vi "Wait for Operation Complete.vi"(8 "error in (no error)":errorcluster, 10 "Timeout (10000 ms)":u32=10000, 11 "VISA resource name":refnum<visa-resource-name>) -> (0 "error out":errorcluster, 3 "VISA resource name out":refnum<visa-resource-name>)   [LabVIEW 2018, in "Keithley 24XX.lvlib"]
doc: "Waits for an operation to complete. This is useful for synchronizing instrument code with other code.\n\n<B>Note:</B> When taking measurements, this VI will hold until the instrument has armed and triggered all of the times specified in Configure Multipoint. This VI won't function correctly if the triggering has occured but the instrument is set to arm after those triggered measurements have finished.\n\nUse this VI only with other low-level VIs. The high-level VIs automatically incorporate this functionality. This VI does not check the instrument status. If you want to check the instrument status, call the Error Query VI at the conclusion of the sequence."
uses:
  Keithley 24XX.lvlib
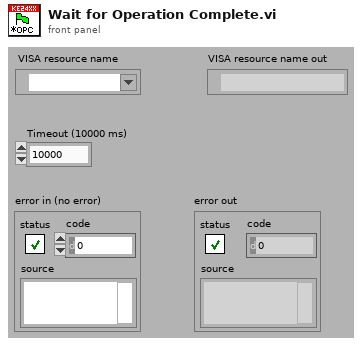
[diagram p1: front panel]
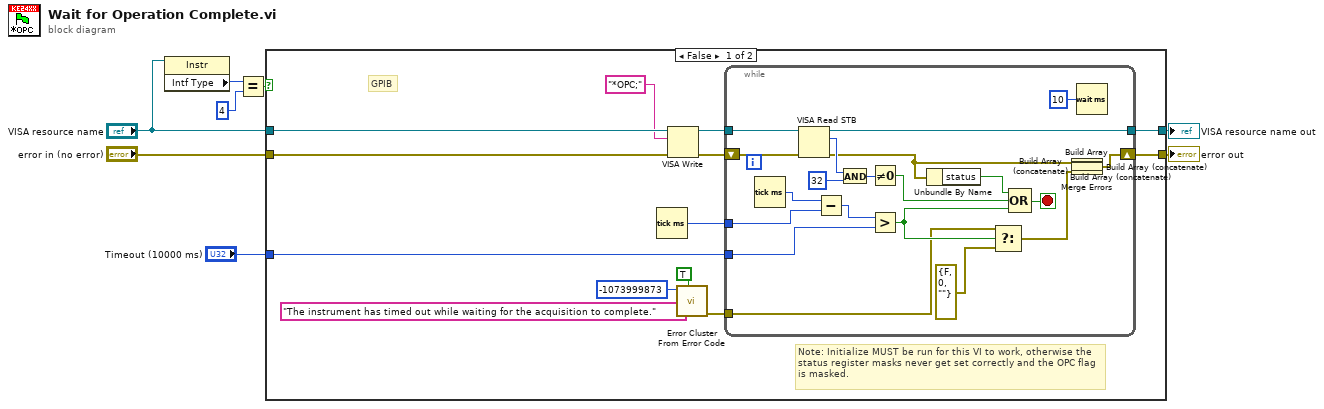
[diagram p0: block diagram]
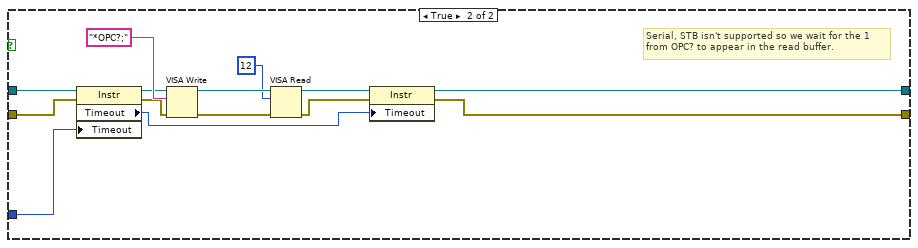
[diagram p2: hidden frame]
diagram:
  n1 = property class="Instr"(reference="VISA resource name") -> ("Intf Type"=w3:u16)  [unwired: 1 in, 2 out]
  n2 = Equal?(x=w3, y=u16 4) -> (x = y?=w4:bool)
  n3 = case shown="False" w4 {
    tunnel: "VISA resource name" -> [w21 w55]
    tunnel: "error in (no error)" -> [w20 w50]
    tunnel: [w17 w46] -> w7
    tunnel: [w16 w51] -> w6
    tunnel: "Timeout (10000 ms)" -> [w9 w54]
    frame False {
      # "GPIB"
      # "Note: Initialize MUST be run for this VI to work, otherwise the status register masks never get set correctly and the OPC flag is masked."
      n4 = Tick Count (ms)() -> (millisecond timer value=w14:u32)
      n5 = VISA Write(VISA resource name=w21, write buffer="*OPC;", error in (no error)=w20) -> (VISA resource name out=w19:refnum<visa-resource-name>, error out=w18:errorcluster)  [unwired: 1 out]
      n6 = call <vilib>:"Error Cluster From Error Code.vi"("show call chain? (False)"=TRUE, "error message (\"\")"="The instrument has timed out while waiting for the acquisition to complete." ("error message (\"\")"), "error code (0)"=-1073999873) -> ("error out"=w10:errorcluster)  [unwired: 6 in]
      n7 = while {
        tunnel: w19 -> [w45]
        tunnel: [w43] -> w16
        tunnel: w14 -> [w38]
        shift-right: [w30] -> w17
        shift-left: w18 -> [w44]
        tunnel: w10 -> [w33]
        tunnel: w9 -> [w26]
        stop <- w35 stop-if-true
        n8 = Tick Count (ms)() -> (millisecond timer value=w39:u32)
        n9 = VISA Read STB(8:w44, 11:w45) -> (0:w29:errorcluster, 2:w42:u16, 3:w43:refnum<visa-resource-name>)
        n10 = Subtract(x=w39, y=w38) -> (x-y=w37:u32)
        n11 = And(x=w42, y=u16 32) -> (x .and. y?=w40:u16)
        n12 = Not Equal To 0?(x=w40) -> (x != 0?=w36:bool)
        n13 = Greater?(x=w37, y=w26) -> (0:w34:bool)
        n14 = Unbundle By Name(w29) -> ("status"=w28:bool)
        n15 = Select(t=w33, s=w34, f=errorcluster {"status"=FALSE, "code"=0, "source"=""}) -> (s? t:f=w31:errorcluster)
        n16 = Compound Arithmetic op=OR(w28, w36, w34) -> (w35:bool)
        n17 = Build Array(w29, w31) -> (w25:errorcluster[])
        n18 = Build Array (concatenate)(w25) -> (w24:errorcluster[])
        n19 = Build Array (concatenate)(w24) -> (w23:errorcluster[])
        n20 = Build Array (concatenate)(w23) -> (w22:errorcluster[])
        n21 = Merge Errors(w22) -> (w30:errorcluster)
        n22 = Wait (ms)(milliseconds to wait=u32 10) -> ()  [unwired: 1 out]
      }
    }
    frame True {
      # "Serial, STB isn't supported so we wait for the 1 \nfrom OPC? to appear in the read buffer."
      n23 = property class="Instr"(reference=w55, error in=w50, "Timeout"=w54) -> (reference out=w49:refnum<visa-resource-name>, error out=w48:errorcluster, "Timeout"=w53:u32)
      n24 = VISA Write(VISA resource name=w49, write buffer="*OPC?;", error in (no error)=w48) -> (VISA resource name out=w57:refnum<visa-resource-name>, error out=w58:errorcluster)  [unwired: 1 out]
      n25 = VISA Read(VISA resource name=w57, byte count=u32 12, error in (no error)=w58) -> (VISA resource name out=w52:refnum<visa-resource-name>, error out=w47:errorcluster)  [unwired: 2 out]
      n26 = property class="Instr"(reference=w52, error in=w47, "Timeout"=w53) -> (reference out=w51:refnum<visa-resource-name>, error out=w46:errorcluster)
    }
  }
  "VISA resource name out" <- w6
  "error out" <- w7
